vi "Set Remove App Event.vi"(8 "error in (no error)":errorcluster, 10 "Remove App":refnum<user-event>, 11 "AppDetailPanel in":refnum<class "AppDetailPanel.lvclass">) -> (0 "error out":errorcluster, 3 "AppDetailPanel out":refnum<class "AppDetailPanel.lvclass">)   [LabVIEW 2020, in "PicoG-App.lvlib" / "AppDetailPanel.lvclass"]
uses:
  AppDetailPanel.lvclass
  ViaApp/ViaApp.lvclass
  AppDetailPanel.lvclass/AppDetailPanel.ctl
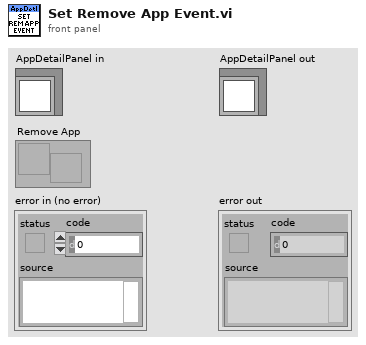
[diagram p1: front panel]
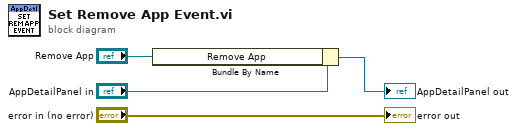
[diagram p0: block diagram]
diagram:
  n1 = Bundle By Name(cluster="AppDetailPanel in", "Remove App"="Remove App") -> (→"AppDetailPanel out":refnum<class "AppDetailPanel.lvclass">)
  "error out" <- "error in (no error)"
